vi "OpenStage_frontpanel.vi"() -> ()   [LabVIEW 2013]
uses:
  <vilib>/Instr/_visa.llb/VISA Configure Serial Port (Instr).vi
panel:
  in  "Beep":bool
  in  "COM Port":refnum<visa-resource-name>="COM3"
  in  "Zero stage":bool
  in  "Goto":bool
  in  "Z":dbl format="%#_6f"
  in  "Y":dbl format="%#_6f"
  in  "X":dbl format="%#_6f"
  in  "stop":bool
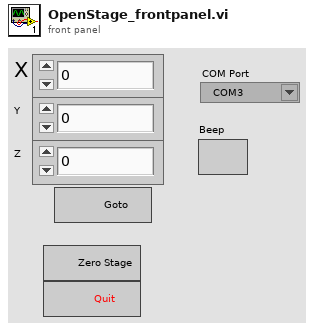
[diagram p1: front panel]
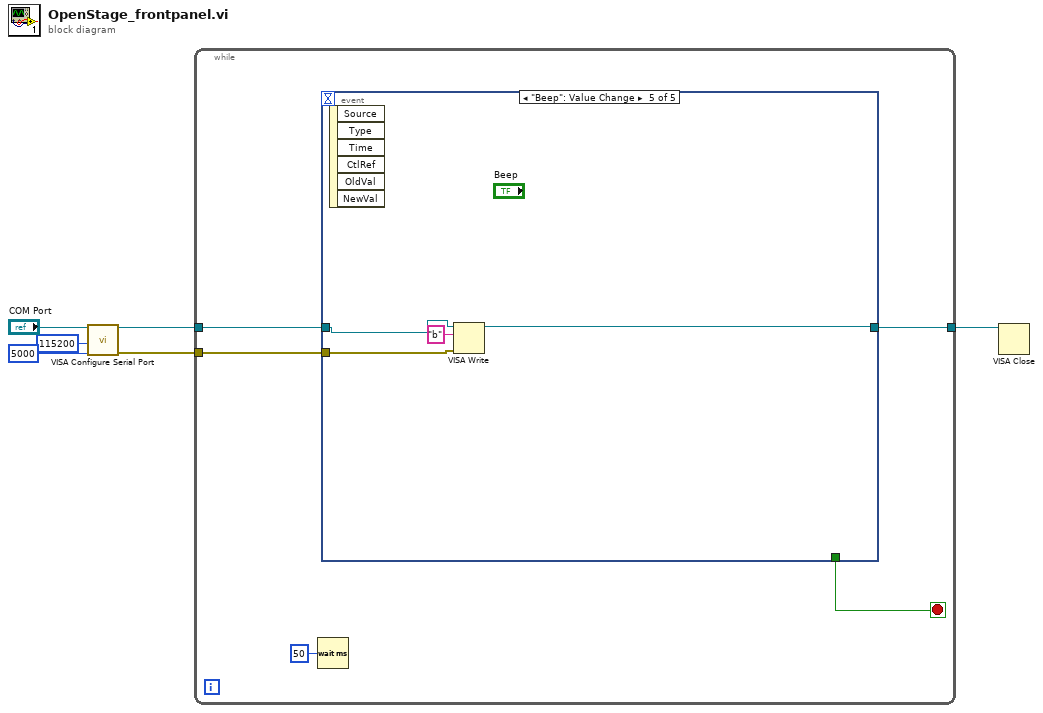
[diagram p0: block diagram]
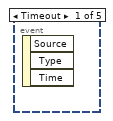
[diagram p2: hidden frame]
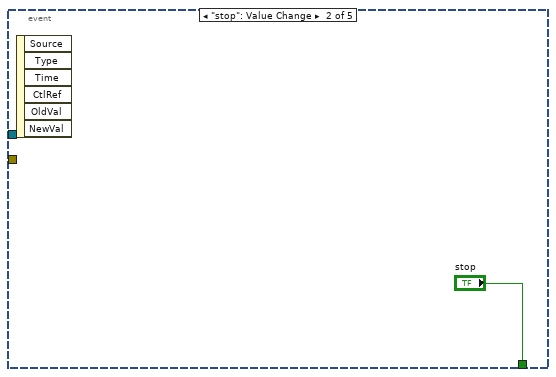
[diagram p3: hidden frame]
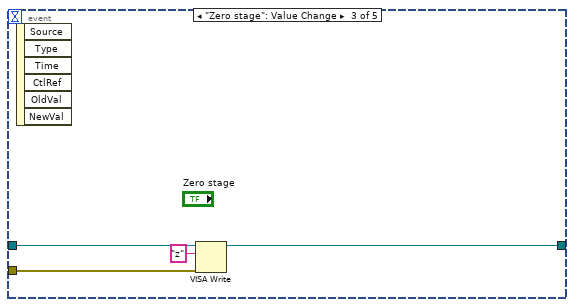
[diagram p4: hidden frame]
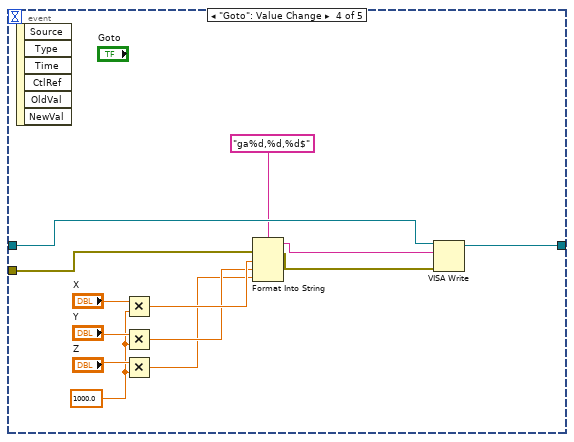
[diagram p5: hidden frame]
diagram:
  n1 = call-poly "VISA Configure Serial Port"("VISA resource name"="COM Port", "timeout (10sec)"=u32 5000, "baud rate (9600)"=u32 115200) -> ("VISA resource name out"=w3:refnum<visa-resource-name>, "error out"=w4:errorcluster)  [unwired: 11 in]
  n2 = while {
    tunnel: w4 -> [w8]
    tunnel: w3 -> [w7]
    tunnel: [w10] -> w2
    stop <- w11 stop-if-true
    n3 = Wait (ms)(milliseconds to wait=u32 50) -> ()  [unwired: 1 out]
    n4 = event shown="[4] \"Beep\": Value Change" {
      selector: _ -> [_ _ _ _ _]
      dyn-events: _ -> [_ _ _ _ _]
      timeout: _ -> [_ _ _ _ _]
      tunnel: [_ "stop" _ _ _] -> w11
      tunnel: w8 -> [_ _ w15 w21 w31]
      tunnel: w7 -> [_ _ w16 w19 w32]
      tunnel: [_ _ w14 w29 w30] -> w10
      event Timeout {
        n5 = event-data() -> ()  [unwired: 1 in, 3 out]
      }
      event "stop": Value Change {
        n6 = event-data() -> ()  [unwired: 1 in, 6 out]
      }
      event "Zero stage": Value Change {
        n7 = event-data() -> ()  [unwired: 1 in, 6 out]
        n8 = VISA Write(VISA resource name=w16, write buffer="z", error in (no error)=w15) -> (VISA resource name out=w14:refnum<visa-resource-name>)  [unwired: 2 out]
      }
      event "Goto": Value Change {
        w25 = 1000.0
        n9 = event-data() -> ()  [unwired: 1 in, 6 out]
        n10 = Multiply(x="X", y=w25) -> (x*y=w24:dbl)
        n11 = Multiply(x="Y", y=w25) -> (x*y=w23:dbl)
        n12 = Multiply(x="Z", y=w25) -> (x*y=w22:dbl)
        n13 = Format Into String(format string="ga%d,%d,%d$", error in=w21, w24, w23, w22) -> (resulting string=w18:string, error out=w20:errorcluster)  [unwired: 1 in]
        n14 = VISA Write(VISA resource name=w19, write buffer=w18, error in (no error)=w20) -> (VISA resource name out=w29:refnum<visa-resource-name>)  [unwired: 2 out]
      }
      event "Beep": Value Change {
        n15 = event-data() -> ()  [unwired: 1 in, 6 out]
        n16 = VISA Write(VISA resource name=w32, write buffer="b", error in (no error)=w31) -> (VISA resource name out=w30:refnum<visa-resource-name>)  [unwired: 2 out]
      }
    }
  }
  n17 = VISA Close(VISA resource name=w2) -> ()  [unwired: 1 in, 1 out]
